vi "contolGroundAxisAutoOnTarget.vi"(7 "Set":bool, 8 "error in":errorcluster, 9 "enable":bool, 10 "axis in":u8, 11 "connection ID":i32) -> (0 "error out":errorcluster, 1 "enable out":bool, 2 "axis out":u8, 3 "connection ID":i32)   [LabVIEW 2016]
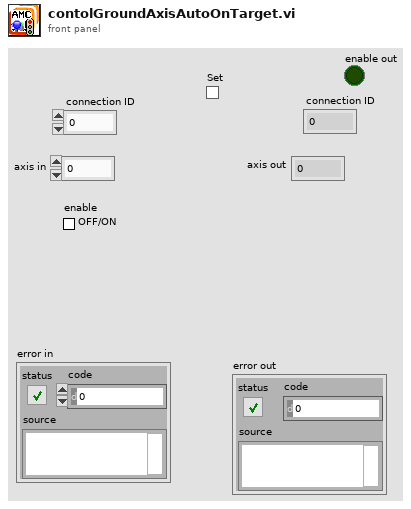
[diagram p1: front panel]
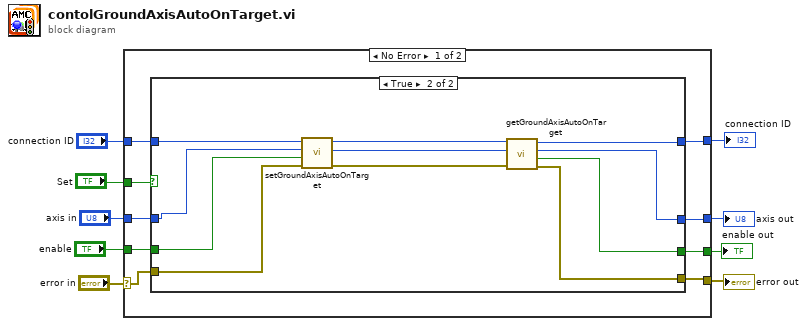
[diagram p0: block diagram]
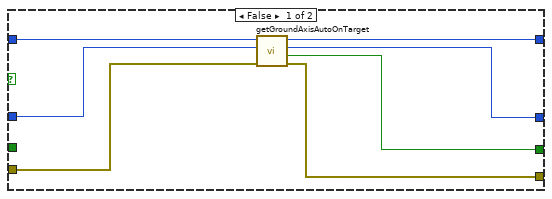
[diagram p2: hidden frame]
diagram:
  n1 = case shown="No Error" "error in" {
    selector: "error in" -> [w11 w40]
    tunnel: "axis in" -> [w16 w39]
    tunnel: [w12 w40] -> w8
    tunnel: [w14 w39] -> w7
    tunnel: [w13 w37] -> w1
    tunnel: "Set" -> [w17 _]
    tunnel: [w15 w38] -> w5
    tunnel: "connection ID" -> [w18 w38]
    tunnel: "enable" -> [w10 w37]
    frame No Error {
      n2 = case shown="True" w17 {
        tunnel: [w24 w31] -> w15
        tunnel: w18 -> [w25 w36]
        tunnel: w16 -> [w21 w34]
        tunnel: [w20 w27] -> w14
        tunnel: [w22 w29] -> w12
        tunnel: [w19 w26] -> w13
        tunnel: w11 -> [w23 w35]
        tunnel: w10 -> [_ w33]
        frame False {
          n3 = call "getGroundAxisAutoOnTarget.vi"("error in"=w23, "axis"=w21, "connection ID"=w25) -> ("error out"=w22:errorcluster, "value"=w19:bool, "axis_out"=w20:i32, "connection ID"=w24:i32)  [unwired: 5 in]
        }
        frame True {
          n4 = call "setGroundAxisAutoOnTarget.vi"("error in"=w35, "enabled"=w33, "axis"=w34, "connection ID"=w36) -> ("error out"=w30:errorcluster, "axis_out"=w28:i32, "connection ID"=w32:i32)  [unwired: 5 in]
          n5 = call "getGroundAxisAutoOnTarget.vi"("error in"=w30, "axis"=w28, "connection ID"=w32) -> ("error out"=w29:errorcluster, "value"=w26:bool, "axis_out"=w27:i32, "connection ID"=w31:i32)  [unwired: 5 in]
        }
      }
    }
    frame Error {
    }
  }
  "error out" <- w8
  "axis out" <- w7
  "connection ID" <- w5
  "enable out" <- w1
